vi "benchmark-tagContainer.vi"() -> (3 "write":dbl[](array[numeric])=[3.499321937561036e-05, 1.2534141540527342e-06, 6.518125534057617e-07, 1.403627395629883e-05, 0.00020125420093536383] caption="average" format="%#_6p")   [LabVIEW 2017]
uses:
  c133460f-0aec-4b14-aa01-684956f011bf.vi
  679e9543-87f0-4a91-8f0b-568c5a8b50fd.vi
  TagContainer/_Support/_NameCacher.vi
  TagContainer/_Support/_datatypeChecker.vi
  TagContainer/_Support/_Ref To DVR.vi
  <vilib>/Utility/Data Type/Get Type Information.vi
  <vilib>/Utility/error.llb/Trim Whitespace.vi
  TagContainer/TagContainer.lvlib
panel:
  out "error out":errorcluster
  in  "group name in (Untitled)":string="add changelock and globalchangetimestamp"
  out "length":i32=1170
  out "unit (ms)":cluster{dbl[]}[](graph)=[{[3.508806228637695e-05, 3.5092830657958984e-05, 3.508806228637695e-05, 3.509044647216797e-05, 3.509759902954102e-05, 3.5092830657958984e-05, 3.5092830657958984e-05, 3.509044647216797e-05, 3.5092830657958984e-05, 3.5092830657958984e-05, 3.509044647216797e-05, 3.509521484375e-05, 3.5092830657958984e-05, 3.508806228637695e-05, 3.509044647216797e-05, 3.5092830657958984e-05, 3.509044647216797e-05, 3.508806228637695e-05, 3.5092830657958984e-05, 3.5092830657958984e-05, 3.509521484375e-05, 3.5092830657958984e-05, 3.5092830657958984e-05, 3.508806228637695e-05, 3.509044647216797e-05, 3.5092830657958984e-05, 3.5092830657958984e-05, 3.5092830657958984e-05, 3.5092830657958984e-05, 3.5092830657958984e-05, 3.5092830657958984e-05, 3.5092830657958984e-05, 3.509044647216797e-05, 3.5092830657958984e-05, 3.509044647216797e-05, 3.509759902954102e-05, 3.509521484375e-05, 3.509521484375e-05, 3.5092830657958984e-05, 3.5092830657958984e-05, 3.5092830657958984e-05, 3.5092830657958984e-05, 3.5092830657958984e-05, 3.5092830657958984e-05, 3.5092830657958984e-05, 3.508806228637695e-05, 3.5092830657958984e-05, 3.5092830657958984e-05, 3.5092830657958984e-05, 3.007650375366211e-05, 3.5092830657958984e-05, 3.509044647216797e-05, 3.509044647216797e-05, 3.508806228637695e-05, 3.509044647216797e-05, 3.508806228637695e-05, 3.509044647216797e-05, 3.5092830657958984e-05, 3.509044647216797e-05, 3.508806228637695e-05, 3.5092830657958984e-05, 3.5092830657958984e-05, 3.509044647216797e-05, 3.509044647216797e-05, 3.5092830657958984e-05, 3.5092830657958984e-05, 3.5092830657958984e-05, 4.024505615234375e-05, 3.5092830657958984e-05, 3.5092830657958984e-05, 3.5092830657958984e-05, 3.5092830657958984e-05, 3.509044647216797e-05, 3.5092830657958984e-05, 3.509044647216797e-05, 3.5092830657958984e-05, 3.5092830657958984e-05, 3.5092830657958984e-05, 3.5092830657958984e-05, 3.008127212524414e-05, 3.0078887939453124e-05, 3.509044647216797e-05, 3.5092830657958984e-05, 3.509044647216797e-05, 3.5092830657958984e-05, 3.508806228637695e-05, 3.508806228637695e-05, 3.5092830657958984e-05, 3.509044647216797e-05, 3.509521484375e-05, 3.509521484375e-05, 3.509759902954102e-05, 3.5092830657958984e-05, 3.5092830657958984e-05, 3.508806228637695e-05, 3.509521484375e-05, 3.509759902954102e-05, 3.509044647216797e-05, 3.5092830657958984e-05, 3.5092830657958984e-05]}, {[0.0, 0.0, 0.0, 0.0, 0.0, 0.0, 0.0, 0.0, 0.0, 0.0, 0.0, 0.0, 0.0, 0.0, 0.0, 5.011558532714844e-06, 5.016326904296875e-06, 0.0, 0.0, 0.0, 0.0, 5.01394271850586e-06, 0.0, 0.0, 5.011558532714844e-06, 5.011558532714844e-06, 0.0, 0.0, 0.0, 0.0, 0.0, 5.016326904296875e-06, 0.0, 0.0, 0.0, 5.011558532714844e-06, 5.011558532714844e-06, 0.0, 5.016326904296875e-06, 0.0, 0.0, 5.011558532714844e-06, 0.0, 5.018711090087891e-06, 0.0, 0.0, 0.0, 0.0, 0.0, 5.016326904296875e-06, 5.016326904296875e-06, 0.0, 0.0, 0.0, 0.0, 0.0, 0.0, 5.016326904296875e-06, 0.0, 0.0, 5.011558532714844e-06, 0.0, 5.01394271850586e-06, 0.0, 0.0, 0.0, 0.0, 5.011558532714844e-06, 5.016326904296875e-06, 0.0, 5.011558532714844e-06, 5.011558532714844e-06, 0.0, 0.0, 0.0, 5.011558532714844e-06, 0.0, 0.0, 0.0, 5.016326904296875e-06, 5.01394271850586e-06, 0.0, 0.0, 5.01394271850586e-06, 0.0, 0.0, 0.0, 0.0, 0.0, 0.0, 5.0091743469238285e-06, 0.0, 0.0, 0.0, 0.0, 0.0, 0.0, 0.0, 0.0, 0.0]}, {[0.0, 0.0, 0.0, 0.0, 0.0, 0.0, 5.016326904296875e-06, 0.0, 0.0, 0.0, 0.0, 0.0, 5.016326904296875e-06, 0.0, 0.0, 0.0, 0.0, 5.01394271850586e-06, 0.0, 0.0, 0.0, 0.0, 0.0, 0.0, 0.0, 0.0, 5.016326904296875e-06, 0.0, 0.0, 0.0, 0.0, 0.0, 0.0, 0.0, 5.016326904296875e-06, 0.0, 0.0, 0.0, 0.0, 0.0, 0.0, 0.0, 0.0, 0.0, 0.0, 0.0, 0.0, 0.0, 5.011558532714844e-06, 0.0, 0.0, 0.0, 0.0, 0.0, 0.0, 5.016326904296875e-06, 0.0, 0.0, 0.0, 0.0, 0.0, 5.016326904296875e-06, 0.0, 0.0, 0.0, 0.0, 0.0, 0.0, 0.0, 0.0, 0.0, 0.0, 5.011558532714844e-06, 5.011558532714844e-06, 0.0, 0.0, 0.0, 0.0, 0.0, 0.0, 0.0, 5.0091743469238285e-06, 0.0, 0.0, 0.0, 0.0, 0.0, 0.0, 5.01394271850586e-06, 0.0, 0.0, 0.0, 0.0, 0.0, 0.0, 0.0, 5.011558532714844e-06, 0.0, 0.0, 0.0]}, {[0.0, 0.0, 5.016326904296875e-06, 5.01394271850586e-06, 0.0, 0.0, 0.0, 0.0, 5.011558532714844e-06, 5.016326904296875e-06, 5.01394271850586e-06, 5.011558532714844e-06, 0.0, 5.01394271850586e-06, 5.01394271850586e-06, 5.01394271850586e-06, 5.011558532714844e-06, 5.01394271850586e-06, 5.011558532714844e-06, 5.011558532714844e-06, 1.0023117065429687e-05, 5.01394271850586e-06, 5.011558532714844e-06, 5.016326904296875e-06, 5.016326904296875e-06, 5.011558532714844e-06, 5.011558532714844e-06, 1.0023117065429687e-05, 1.0023117065429687e-05, 1.0023117065429687e-05, 1.0023117065429687e-05, 5.011558532714844e-06, 1.0025501251220702e-05, 1.0023117065429687e-05, 5.011558532714844e-06, 1.0023117065429687e-05, 1.0025501251220702e-05, 1.0023117065429687e-05, 1.0023117065429687e-05, 1.5039443969726562e-05, 1.5039443969726562e-05, 1.002788543701172e-05, 1.5034675598144532e-05, 1.0020732879638672e-05, 1.5037059783935547e-05, 1.5039443969726562e-05, 1.5037059783935547e-05, 1.5039443969726562e-05, 1.0025501251220702e-05, 1.5039443969726562e-05, 1.0023117065429687e-05, 1.5037059783935547e-05, 1.5039443969726562e-05, 1.5041828155517579e-05, 2.0053386688232422e-05, 1.5041828155517579e-05, 1.5041828155517579e-05, 1.5034675598144532e-05, 1.5039443969726562e-05, 1.5039443969726562e-05, 1.5039443969726562e-05, 1.5034675598144532e-05, 1.5039443969726562e-05, 1.5041828155517579e-05, 2.0053386688232422e-05, 2.0051002502441405e-05, 2.0051002502441405e-05, 1.5056133270263672e-05, 1.5034675598144532e-05, 2.0053386688232422e-05, 2.0051002502441405e-05, 2.0051002502441405e-05, 2.0053386688232422e-05, 2.005577087402344e-05, 2.5064945220947265e-05, 2.0053386688232422e-05, 2.0051002502441405e-05, 2.0051002502441405e-05, 2.506256103515625e-05, 2.0051002502441405e-05, 2.0051002502441405e-05, 2.005577087402344e-05, 2.506732940673828e-05, 2.005577087402344e-05, 2.506256103515625e-05, 2.506732940673828e-05, 2.5069713592529298e-05, 2.506732940673828e-05, 2.506256103515625e-05, 2.5060176849365234e-05, 2.506732940673828e-05, 2.506256103515625e-05, 2.506256103515625e-05, 3.007650375366211e-05, 3.008127212524414e-05, 2.5064945220947265e-05, 2.506256103515625e-05, 2.5064945220947265e-05, 3.008127212524414e-05, 3.0074119567871094e-05]}, {[5.011558532714844e-06, 1.002788543701172e-05, 1.002788543701172e-05, 1.5034675598144532e-05, 2.506256103515625e-05, 2.506256103515625e-05, 3.007650375366211e-05, 3.5092830657958984e-05, 3.509044647216797e-05, 4.010438919067383e-05, 4.511594772338867e-05, 4.511594772338867e-05, 5.514621734619141e-05, 5.514383316040039e-05, 6.015777587890625e-05, 6.0155391693115235e-05, 6.517410278320313e-05, 7.018327713012695e-05, 8.021116256713867e-05, 8.020877838134766e-05, 8.020877838134766e-05, 9.023427963256837e-05, 9.525299072265625e-05, 9.524822235107422e-05, 0.00010048389434814453, 0.00010527610778808594, 0.00011028766632080078, 0.00011029243469238282, 0.00011530399322509766, 0.0001203155517578125, 0.0001203155517578125, 0.00013034105300903322, 0.00013535499572753907, 0.00013535737991333008, 0.0001403641700744629, 0.00014036893844604492, 0.0001503920555114746, 0.0001503920555114746, 0.0001554083824157715, 0.00015540361404418944, 0.00016041994094848633, 0.00017044782638549804, 0.00017044782638549804, 0.00018047094345092775, 0.00018047571182250977, 0.0001854872703552246, 0.00019049882888793945, 0.00019049882888793945, 0.00020052671432495118, 0.00019550800323486328, 0.00020554065704345704, 0.00020554065704345704, 0.00021055221557617188, 0.00021556377410888672, 0.00021556615829467773, 0.00022057533264160155, 0.0002255868911743164, 0.0002306056022644043, 0.000240633487701416, 0.000240631103515625, 0.00024062871932983398, 0.00024564504623413085, 0.0002506566047668457, 0.0002556657791137695, 0.00025567054748535154, 0.00026067972183227536, 0.0002656960487365723, 0.0002706313133239746, 0.000275723934173584, 0.00027571916580200196, 0.000275723934173584, 0.00028073787689208984, 0.00028574705123901367, 0.0002907609939575195, 0.0002957749366760254, 0.0003007864952087402, 0.00030580043792724607, 0.000310816764831543, 0.0003158235549926758, 0.0003184247016906738, 0.0003208446502685547, 0.00033086299896240235, 0.00033086538314819336, 0.00034089088439941405, 0.00034089326858520507, 0.0003408956527709961, 0.00035091400146484373, 0.00035092115402221677, 0.00035593271255493166, 0.00035593271255493166, 0.0003609395027160645, 0.00036596059799194337, 0.0003709721565246582, 0.0003709745407104492, 0.0003809952735900879, 0.00038600683212280273, 0.0003910255432128906, 0.0003910231590270996, 0.00039603471755981443, 0.00039603710174560545]}]
  out "outside":i32=99
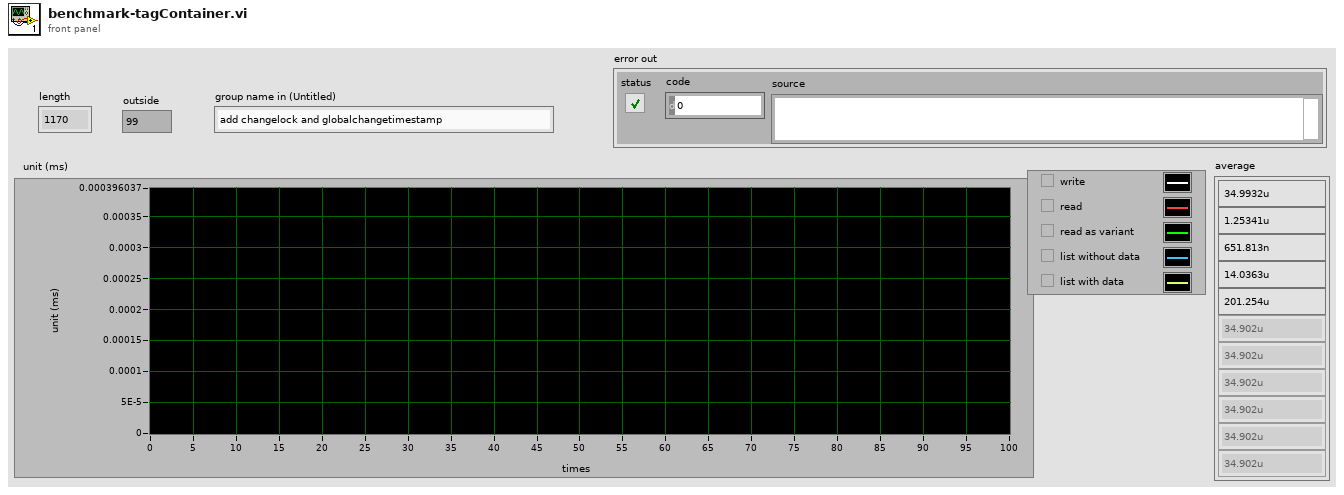
[diagram p1: front panel]
types:
  T1 = enum16{"open", "open or create", "create or replace", "create", "open (read-only)"}
  T2 = cluster{"error constant":errorcluster, "error constant 2":errorcluster, "error constant 3":errorcluster, "error constant 4":errorcluster, "error constant 5":errorcluster, "error constant 6":errorcluster, "error constant 7":errorcluster, "error constant 8":errorcluster, "error constant 9":errorcluster, "error constant 10":errorcluster, "error constant 11":errorcluster, "error constant 12":errorcluster, "error constant 13":errorcluster, "error constant 14":errorcluster, "error constant 15":errorcluster, "error constant 16":errorcluster, "error constant 17":errorcluster, "error constant 18":errorcluster, "error constant 19":errorcluster, "error constant 20":errorcluster, "error constant 21":errorcluster, "error constant 22":errorcluster, "error constant 23":errorcluster, "error constant 24":errorcluster, "error constant 25":errorcluster, "error constant 26":errorcluster, "error constant 27":errorcluster, "error constant 28":errorcluster, "error constant 29":errorcluster, "error constant 30":errorcluster, "error constant 31":errorcluster, "error constant 32":errorcluster, "error constant 33":errorcluster, "error constant 34":errorcluster, "error constant 35":errorcluster, "error constant 36":errorcluster, "error constant 37":errorcluster, "error constant 38":errorcluster, "error constant 39":errorcluster, "error constant 40":errorcluster, "error constant 41":errorcluster, "error constant 42":errorcluster, "error constant 43":errorcluster, "error constant 44":errorcluster, "error constant 45":errorcluster, "error constant 46":errorcluster, "error constant 47":errorcluster, "error constant 48":errorcluster, "error constant 49":errorcluster, "error constant 50":errorcluster, "error constant 51":errorcluster, "error constant 52":errorcluster, "error constant 53":errorcluster, "error constant 54":errorcluster, "error constant 55":errorcluster, "error constant 56":errorcluster, "error constant 57":errorcluster, "error constant 58":errorcluster, "error constant 59":errorcluster, "error constant 60":errorcluster, "error constant 61":errorcluster, "error constant 62":errorcluster, "error constant 63":errorcluster, "error constant 64":errorcluster, "error constant 65":errorcluster, cluster{"error constant":errorcluster, "error constant 2":errorcluster, "error constant 3":errorcluster, "error constant 4":errorcluster, "error constant 5":errorcluster, "error constant 6":errorcluster, "error constant 7":errorcluster, "error constant 8":errorcluster, "error constant 9":errorcluster, "error constant 10":errorcluster, "error constant 11":errorcluster, "error constant 12":errorcluster, "error constant 13":errorcluster, "error constant 14":errorcluster, "error constant 15":errorcluster, "error constant 16":errorcluster, "error constant 17":errorcluster, "error constant 18":errorcluster, "error constant 19":errorcluster, "error constant 20":errorcluster, "error constant 21":errorcluster, "error constant 22":errorcluster, "error constant 23":errorcluster, "error constant 24":errorcluster, "error constant 25":errorcluster, "error constant 26":errorcluster, "error constant 27":errorcluster, "error constant 28":errorcluster, "error constant 29":errorcluster, "error constant 30":errorcluster, "error constant 31":errorcluster, "error constant 32":errorcluster, "error constant 33":errorcluster, "error constant 34":errorcluster, "error constant 35":errorcluster, "error constant 36":errorcluster, "error constant 37":errorcluster, "error constant 38":errorcluster, "error constant 39":errorcluster, "error constant 40":errorcluster, "error constant 41":errorcluster, "error constant 42":errorcluster, "error constant 43":errorcluster, "error constant 44":errorcluster, "error constant 45":errorcluster, "error constant 46":errorcluster, "error constant 47":errorcluster, "error constant 48":errorcluster, "error constant 49":errorcluster, "error constant 50":errorcluster, "error constant 51":errorcluster, "error constant 52":errorcluster, "error constant 53":errorcluster, "error constant 54":errorcluster, "error constant 55":errorcluster, "error constant 56":errorcluster, "error constant 57":errorcluster, "error constant 58":errorcluster, "error constant 59":errorcluster, "error constant 60":errorcluster, "error constant 61":errorcluster, "error constant 62":errorcluster, "error constant 63":errorcluster, "error constant 64":errorcluster, "error constant 65":errorcluster}}
  T3 = typedef "TagContainer.lvlib/TagContainer.ctl" = refnum<k1>
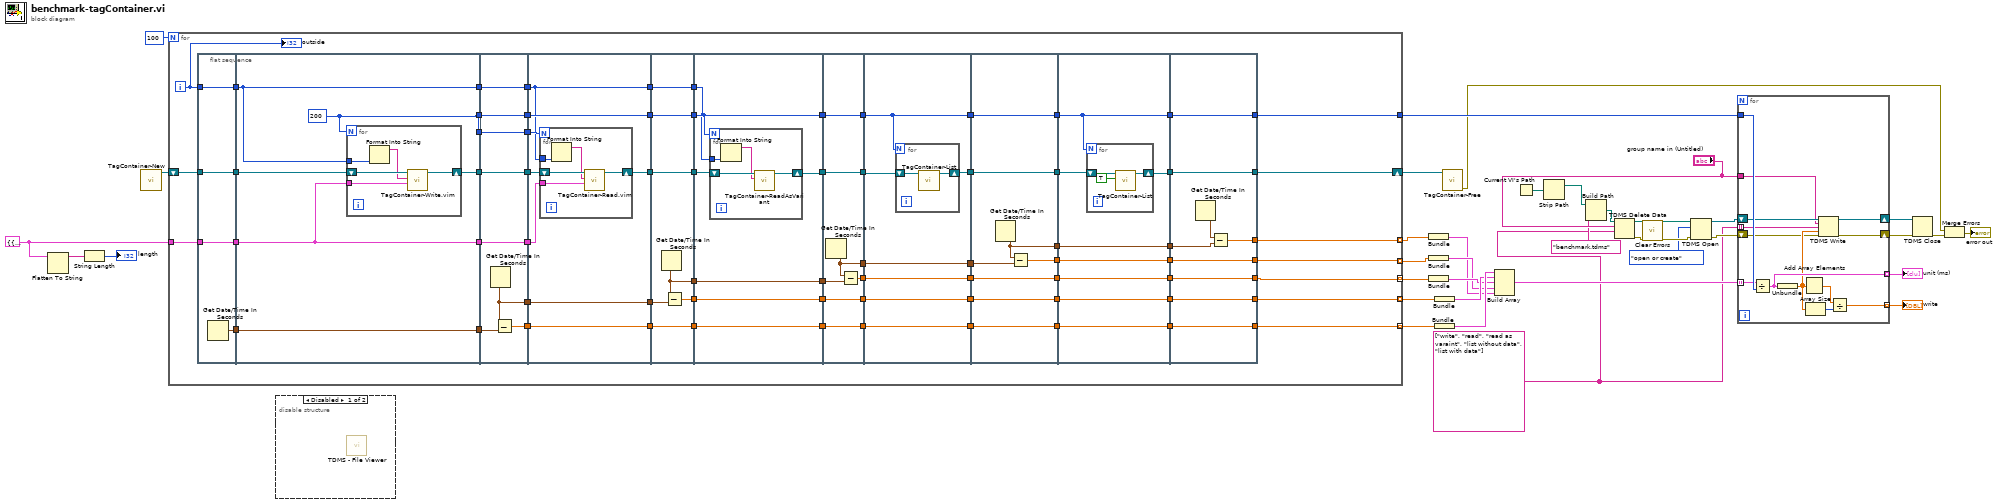
[diagram p0: block diagram]
diagram:
  w3 = string[] ["write", "read", "read as varaint", "list without data", "list with data"]
  w33 = T2 {"error constant"={"status"=FALSE, "code"=0, "source"=""}, "error constant 2"={"status"=FALSE, "code"=0, "source"=""}, "error constant 3"={"status"=FALSE, "code"=0, "source"=""}, "error constant 4"={"status"=FALSE, "code"=0, "source"=""}, "error constant 5"={"status"=FALSE, "code"=0, "source"=""}, "error constant 6"={"status"=FALSE, "code"=0, "source"=""}, "error constant 7"={"status"=FALSE, "code"=0, "source"=""}, "error constant 8"={"status"=FALSE, "code"=0, "source"=""}, "error constant 9"={"status"=FALSE, "code"=0, "source"=""}, "error constant 10"={"status"=FALSE, "code"=0, "source"=""}, "error constant 11"={"status"=FALSE, "code"=0, "source"=""}, "error constant 12"={"status"=FALSE, "code"=0, "source"=""}, "error constant 13"={"status"=FALSE, "code"=0, "source"=""}, "error constant 14"={"status"=FALSE, "code"=0, "source"=""}, "error constant 15"={"status"=FALSE, "code"=0, "source"=""}, "error constant 16"={"status"=FALSE, "code"=0, "source"=""}, "error constant 17"={"status"=FALSE, "code"=0, "source"=""}, "error constant 18"={"status"=FALSE, "code"=0, "source"=""}, "error constant 19"={"status"=FALSE, "code"=0, "source"=""}, "error constant 20"={"status"=FALSE, "code"=0, "source"=""}, "error constant 21"={"status"=FALSE, "code"=0, "source"=""}, "error constant 22"={"status"=FALSE, "code"=0, "source"=""}, "error constant 23"={"status"=FALSE, "code"=0, "source"=""}, "error constant 24"={"status"=FALSE, "code"=0, "source"=""}, "error constant 25"={"status"=FALSE, "code"=0, "source"=""}, "error constant 26"={"status"=FALSE, "code"=0, "source"=""}, "error constant 27"={"status"=FALSE, "code"=0, "source"=""}, "error constant 28"={"status"=FALSE, "code"=0, "source"=""}, "error constant 29"={"status"=FALSE, "code"=0, "source"=""}, "error constant 30"={"status"=FALSE, "code"=0, "source"=""}, "error constant 31"={"status"=FALSE, "code"=0, "source"=""}, "error constant 32"={"status"=FALSE, "code"=0, "source"=""}, "error constant 33"={"status"=FALSE, "code"=0, "source"=""}, "error constant 34"={"status"=FALSE, "code"=0, "source"=""}, "error constant 35"={"status"=FALSE, "code"=0, "source"=""}, "error constant 36"={"status"=FALSE, "code"=0, "source"=""}, "error constant 37"={"status"=FALSE, "code"=0, "source"=""}, "error constant 38"={"status"=FALSE, "code"=0, "source"=""}, "error constant 39"={"status"=FALSE, "code"=0, "source"=""}, "error constant 40"={"status"=FALSE, "code"=0, "source"=""}, "error constant 41"={"status"=FALSE, "code"=0, "source"=""}, "error constant 42"={"status"=FALSE, "code"=0, "source"=""}, "error constant 43"={"status"=FALSE, "code"=0, "source"=""}, "error constant 44"={"status"=FALSE, "code"=0, "source"=""}, "error constant 45"={"status"=FALSE, "code"=0, "source"=""}, "error constant 46"={"status"=FALSE, "code"=0, "source"=""}, "error constant 47"={"status"=FALSE, "code"=0, "source"=""}, "error constant 48"={"status"=FALSE, "code"=0, "source"=""}, "error constant 49"={"status"=FALSE, "code"=0, "source"=""}, "error constant 50"={"status"=FALSE, "code"=0, "source"=""}, "error constant 51"={"status"=FALSE, "code"=0, "source"=""}, "error constant 52"={"status"=FALSE, "code"=0, "source"=""}, "error constant 53"={"status"=FALSE, "code"=0, "source"=""}, "error constant 54"={"status"=FALSE, "code"=0, "source"=""}, "error constant 55"={"status"=FALSE, "code"=0, "source"=""}, "error constant 56"={"status"=FALSE, "code"=0, "source"=""}, "error constant 57"={"status"=FALSE, "code"=0, "source"=""}, "error constant 58"={"status"=FALSE, "code"=0, "source"=""}, "error constant 59"={"status"=FALSE, "code"=0, "source"=""}, "error constant 60"={"status"=FALSE, "code"=0, "source"=""}, "error constant 61"={"status"=FALSE, "code"=0, "source"=""}, "error constant 62"={"status"=FALSE, "code"=0, "source"=""}, "error constant 63"={"status"=FALSE, "code"=0, "source"=""}, "error constant 64"={"status"=FALSE, "code"=0, "source"=""}, "error constant 65"={"status"=FALSE, "code"=0, "source"=""}, {"error constant"={"status"=FALSE, "code"=0, "source"=""}, "error constant 2"={"status"=FALSE, "code"=0, "source"=""}, "error constant 3"={"status"=FALSE, "code"=0, "source"=""}, "error constant 4"={"status"=FALSE, "code"=0, "source"=""}, "error constant 5"={"status"=FALSE, "code"=0, "source"=""}, "error constant 6"={"status"=FALSE, "code"=0, "source"=""}, "error constant 7"={"status"=FALSE, "code"=0, "source"=""}, "error constant 8"={"status"=FALSE, "code"=0, "source"=""}, "error constant 9"={"status"=FALSE, "code"=0, "source"=""}, "error constant 10"={"status"=FALSE, "code"=0, "source"=""}, "error constant 11"={"status"=FALSE, "code"=0, "source"=""}, "error constant 12"={"status"=FALSE, "code"=0, "source"=""}, "error constant 13"={"status"=FALSE, "code"=0, "source"=""}, "error constant 14"={"status"=FALSE, "code"=0, "source"=""}, "error constant 15"={"status"=FALSE, "code"=0, "source"=""}, "error constant 16"={"status"=FALSE, "code"=0, "source"=""}, "error constant 17"={"status"=FALSE, "code"=0, "source"=""}, "error constant 18"={"status"=FALSE, "code"=0, "source"=""}, "error constant 19"={"status"=FALSE, "code"=0, "source"=""}, "error constant 20"={"status"=FALSE, "code"=0, "source"=""}, "error constant 21"={"status"=FALSE, "code"=0, "source"=""}, "error constant 22"={"status"=FALSE, "code"=0, "source"=""}, "error constant 23"={"status"=FALSE, "code"=0, "source"=""}, "error constant 24"={"status"=FALSE, "code"=0, "source"=""}, "error constant 25"={"status"=FALSE, "code"=0, "source"=""}, "error constant 26"={"status"=FALSE, "code"=0, "source"=""}, "error constant 27"={"status"=FALSE, "code"=0, "source"=""}, "error constant 28"={"status"=FALSE, "code"=0, "source"=""}, "error constant 29"={"status"=FALSE, "code"=0, "source"=""}, "error constant 30"={"status"=FALSE, "code"=0, "source"=""}, "error constant 31"={"status"=FALSE, "code"=0, "source"=""}, "error constant 32"={"status"=FALSE, "code"=0, "source"=""}, "error constant 33"={"status"=FALSE, "code"=0, "source"=""}, "error constant 34"={"status"=FALSE, "code"=0, "source"=""}, "error constant 35"={"status"=FALSE, "code"=0, "source"=""}, "error constant 36"={"status"=FALSE, "code"=0, "source"=""}, "error constant 37"={"status"=FALSE, "code"=0, "source"=""}, "error constant 38"={"status"=FALSE, "code"=0, "source"=""}, "error constant 39"={"status"=FALSE, "code"=0, "source"=""}, "error constant 40"={"status"=FALSE, "code"=0, "source"=""}, "error constant 41"={"status"=FALSE, "code"=0, "source"=""}, "error constant 42"={"status"=FALSE, "code"=0, "source"=""}, "error constant 43"={"status"=FALSE, "code"=0, "source"=""}, "error constant 44"={"status"=FALSE, "code"=0, "source"=""}, "error constant 45"={"status"=FALSE, "code"=0, "source"=""}, "error constant 46"={"status"=FALSE, "code"=0, "source"=""}, "error constant 47"={"status"=FALSE, "code"=0, "source"=""}, "error constant 48"={"status"=FALSE, "code"=0, "source"=""}, "error constant 49"={"status"=FALSE, "code"=0, "source"=""}, "error constant 50"={"status"=FALSE, "code"=0, "source"=""}, "error constant 51"={"status"=FALSE, "code"=0, "source"=""}, "error constant 52"={"status"=FALSE, "code"=0, "source"=""}, "error constant 53"={"status"=FALSE, "code"=0, "source"=""}, "error constant 54"={"status"=FALSE, "code"=0, "source"=""}, "error constant 55"={"status"=FALSE, "code"=0, "source"=""}, "error constant 56"={"status"=FALSE, "code"=0, "source"=""}, "error constant 57"={"status"=FALSE, "code"=0, "source"=""}, "error constant 58"={"status"=FALSE, "code"=0, "source"=""}, "error constant 59"={"status"=FALSE, "code"=0, "source"=""}, "error constant 60"={"status"=FALSE, "code"=0, "source"=""}, "error constant 61"={"status"=FALSE, "code"=0, "source"=""}, "error constant 62"={"status"=FALSE, "code"=0, "source"=""}, "error constant 63"={"status"=FALSE, "code"=0, "source"=""}, "error constant 64"={"status"=FALSE, "code"=0, "source"=""}, "error constant 65"={"status"=FALSE, "code"=0, "source"=""}}}
  n1 = Flatten To String(anything=w33) -> (data string=w32:string)  [unwired: 3 in, 2 out]
  n2 = String Length(string=w32) -> (length=→"length":i32)
  n3 = call "TagContainer-New.vi"() -> ("TagContainer"=w35:T3)  [unwired: 10 in, 1 out]
  n4 = for {
    N: 100 -> [_]
    tunnel: [w104] -> w27 mode=indexing
    tunnel: [w103] -> w29
    tunnel: w33 -> [w93]
    shift-right: [w91] -> w34
    shift-left: w35 -> [w92]
    tunnel: [w86] -> w28 mode=indexing
    tunnel: [w73] -> w25 mode=indexing
    tunnel: [w39] -> w24 mode=indexing
    tunnel: [w38] -> w23 mode=indexing
    i -> [w101]
    n5 = flat-sequence {
      tunnel: [w110] -> w106
      tunnel: [w109] -> w96
      tunnel: [w108] -> w95
      tunnel: [w107] -> w94
      tunnel: w92 -> [w109]
      tunnel: w93 -> [w108]
      tunnel: w101 -> [w107]
      tunnel: w106 -> [w116]
      tunnel: [w116] -> w105
      tunnel: [w112] -> w102
      tunnel: [w114] -> w97
      tunnel: w96 -> [w115]
      tunnel: w95 -> [w111]
      tunnel: w94 -> [w113]
      tunnel: [w112] -> w84
      tunnel: [w113] -> w81
      tunnel: [w111] -> w79
      tunnel: w105 -> [w126]
      tunnel: w102 -> [w128]
      tunnel: [w129] -> w100
      tunnel: [w128] -> w99
      tunnel: [w127] -> w98
      tunnel: w97 -> [w127]
      tunnel: [w122] -> w88
      tunnel: w84 -> [w125]
      tunnel: [w125] -> w83
      tunnel: [w124] -> w82
      tunnel: w81 -> [w124]
      tunnel: [w123] -> w80
      tunnel: w79 -> [w123]
      tunnel: w100 -> [w137]
      tunnel: w99 -> [w136]
      tunnel: w98 -> [w134]
      tunnel: [w137] -> w90
      tunnel: [w136] -> w89
      tunnel: w88 -> [w135]
      tunnel: [w135] -> w87
      tunnel: [w133] -> w85
      tunnel: w83 -> [w132]
      tunnel: w82 -> [w130]
      tunnel: w80 -> [w131]
      tunnel: [w130] -> w72
      tunnel: w90 -> [w149]
      tunnel: w89 -> [w146]
      tunnel: w87 -> [w148]
      tunnel: w85 -> [w144]
      tunnel: [w149] -> w71
      tunnel: [w146] -> w70
      tunnel: [w147] -> w69
      tunnel: [w145] -> w68
      tunnel: w72 -> [w145]
      tunnel: [w144] -> w67
      tunnel: [w143] -> w66
      tunnel: w71 -> [w156]
      tunnel: w70 -> [w153]
      tunnel: w69 -> [w155]
      tunnel: [w156] -> w78
      tunnel: [w153] -> w77
      tunnel: [w154] -> w76
      tunnel: [w155] -> w75
      tunnel: [w150] -> w74
      tunnel: w68 -> [w152]
      tunnel: w67 -> [w151]
      tunnel: w66 -> [w150]
      tunnel: w78 -> [w167]
      tunnel: w77 -> [w166]
      tunnel: w76 -> [w165]
      tunnel: w75 -> [w164]
      tunnel: w74 -> [w163]
      tunnel: [w167] -> w65
      tunnel: [w166] -> w64
      tunnel: [w165] -> w63
      tunnel: [w164] -> w62
      tunnel: [w162] -> w61
      tunnel: [w161] -> w55
      tunnel: w65 -> [w174]
      tunnel: w64 -> [w168]
      tunnel: w63 -> [w171]
      tunnel: w62 -> [w173]
      tunnel: w61 -> [w172]
      tunnel: [w174] -> w60
      tunnel: [w168] -> w59
      tunnel: [w170] -> w58
      tunnel: [w173] -> w57
      tunnel: [w172] -> w56
      tunnel: w55 -> [w169]
      tunnel: [w169] -> w54
      tunnel: w60 -> [w184]
      tunnel: w59 -> [w183]
      tunnel: w58 -> [w182]
      tunnel: w57 -> [w181]
      tunnel: w56 -> [w180]
      tunnel: w54 -> [w179]
      tunnel: [w184] -> w53
      tunnel: [w183] -> w52
      tunnel: [w182] -> w51
      tunnel: [w181] -> w50
      tunnel: [w180] -> w49
      tunnel: [w178] -> w48
      tunnel: [w177] -> w41
      tunnel: w53 -> [w192]
      tunnel: w52 -> [w185]
      tunnel: w51 -> [w188]
      tunnel: w50 -> [w191]
      tunnel: w49 -> [w190]
      tunnel: w48 -> [w189]
      tunnel: [w192] -> w47
      tunnel: [w185] -> w46
      tunnel: [w187] -> w45
      tunnel: [w191] -> w44
      tunnel: [w190] -> w43
      tunnel: [w189] -> w42
      tunnel: w41 -> [w186]
      tunnel: [w186] -> w40
      tunnel: [w199] -> w38
      tunnel: [w200] -> w73
      tunnel: [w201] -> w86
      tunnel: [w202] -> w91
      tunnel: [w203] -> w103
      tunnel: [w204] -> w104
      tunnel: w47 -> [w204]
      tunnel: w46 -> [w203]
      tunnel: w45 -> [w202]
      tunnel: w44 -> [w201]
      tunnel: w43 -> [w200]
      tunnel: w42 -> [w199]
      tunnel: w40 -> [w197]
      tunnel: [w196] -> w39
      frame #0 {
        n6 = Get Date/Time In Seconds() -> (seconds since 1Jan1904=w110:timestamp)
      }
      frame #1 {
        w112 = 200
        n7 = for {
          N: w112 -> [_]
          tunnel: w111 -> [w119]
          tunnel: w113 -> [w118]
          shift-right: [w120] -> w114
          shift-left: w115 -> [w121]
          n8 = Format Into String(w118) -> (resulting string=w117:string)  [unwired: 3 in, 1 out]
          n9 = call "TagContainer-Write.vim"("Value"=w119, "name"=w117, "TagContainer"=w121) -> ("TagContainer(dup)"=w120:T3)  [unwired: 7 in, 1 out]
        }
      }
      frame #2 {
        n10 = Get Date/Time In Seconds() -> (seconds since 1Jan1904=w122:timestamp)
        n11 = Subtract(x=w122, y=w126) -> (x-y=w129:dbl)
      }
      frame #3 {
        n12 = for {
          N: w132 -> [_]
          shift-right: [w141] -> w133
          shift-left: w134 -> [w142]
          tunnel: w130 -> [w139]
          tunnel: w131 -> [w138]
          n13 = Format Into String(w139) -> (resulting string=w140:string)  [unwired: 3 in, 1 out]
          n14 = call "TagContainer-Read.vim"("Type"=w138, "name"=w140, "TagContainer"=w142) -> ("TagContainer(dup)"=w141:T3)  [unwired: 3 in, 5 out]
        }
      }
      frame #4 {
        n15 = Get Date/Time In Seconds() -> (seconds since 1Jan1904=w143:timestamp)
        n16 = Subtract(x=w143, y=w148) -> (x-y=w147:dbl)
      }
      frame #5 {
        n17 = for {
          N: w153 -> [_]
          shift-right: [w159] -> w154
          shift-left: w151 -> [w160]
          tunnel: w152 -> [w157]
          n18 = Format Into String(w157) -> (resulting string=w158:string)  [unwired: 3 in, 1 out]
          n19 = call "TagContainer-ReadAsVariant.vi"("name"=w158, "TagContainer"=w160) -> ("TagContainer(dup)"=w159:T3)  [unwired: 4 in, 5 out]
        }
      }
      frame #6 {
        n20 = Get Date/Time In Seconds() -> (seconds since 1Jan1904=w161:timestamp)
        n21 = Subtract(x=w161, y=w163) -> (x-y=w162:dbl)
      }
      frame #7 {
        n22 = for {
          N: w168 -> [_]
          shift-right: [w175] -> w170
          shift-left: w171 -> [w176]
          n23 = call "TagContainer-List.vi"("TagContainer"=w176) -> ("TagContainer(dup)"=w175:T3)  [unwired: 7 in, 3 out]
        }
      }
      frame #8 {
        n24 = Get Date/Time In Seconds() -> (seconds since 1Jan1904=w177:timestamp)
        n25 = Subtract(x=w177, y=w179) -> (x-y=w178:dbl)
      }
      frame #9 {
        n26 = for {
          N: w185 -> [_]
          shift-right: [w194] -> w187
          shift-left: w188 -> [w195]
          n27 = call "TagContainer-List.vi"("with Data?(F)"=TRUE, "TagContainer"=w195) -> ("TagContainer(dup)"=w194:T3)  [unwired: 6 in, 3 out]
        }
      }
      frame #10 {
        n28 = Get Date/Time In Seconds() -> (seconds since 1Jan1904=w198:timestamp)
        n29 = Subtract(x=w198, y=w197) -> (x-y=w196:dbl)
      }
    }
    "outside" <- w101
  }
  n30 = disable-structure shown="Disabled" {
    frame Disabled {
      n31 = call <vilib>:"TDMS - File Viewer.vi"() -> ()  [unwired: 6 in, 2 out]
    }
    frame Enabled {
    }
  }
  n32 = Bundle(w24) -> (w18:cluster{dbl[]})  [unwired: 1 in]
  n33 = Bundle(w23) -> (w19:cluster{dbl[]})  [unwired: 1 in]
  n34 = Bundle(w25) -> (w20:cluster{dbl[]})  [unwired: 1 in]
  n35 = Bundle(w28) -> (w21:cluster{dbl[]})  [unwired: 1 in]
  n36 = Bundle(w27) -> (w22:cluster{dbl[]})  [unwired: 1 in]
  n37 = call "TagContainer-Free.vi"("TagContainer"=w34) -> ("error out"=w5:errorcluster)  [unwired: 10 in]
  n38 = Build Array(w22, w21, w20, w19, w18) -> (w26:cluster{dbl[]}[])
  n39 = Current VI's Path() -> (path=w2:path)
  n40 = Strip Path(path=w2) -> (stripped path=w1:path)  [unwired: 1 out]
  n41 = Build Path(base path=w1, name or relative path="benchmark.tdms") -> (appended path=w10:path)
  n42 = TDMS Delete Data(9:w3, 10:"group name in (Untitled)", 11:w10) -> (0:w12:errorcluster, 3:w11:path)  [unwired: 4 in]
  n43 = call <vilib>:"Clear Errors.vi"("error in (no error)"=w12) -> ("error out"=w8:errorcluster)  [unwired: 5 in, 1 out]
  n44 = TDMS Open(8:w8, 10:T1."open or create" ("operation (0:open)"), 11:w11) -> (0:w15:errorcluster, 3:w14:refnum<k34>)  [unwired: 4 in]
  n45 = for {
    tunnel: [w217] -> w31 mode=indexing
    tunnel: [w212] -> w30 mode=indexing
    tunnel: w29 -> [w214]
    tunnel: w26 -> [w213] mode=indexing
    shift-right: [w210] -> w17
    shift-left: w14 -> [w209]
    shift-right: [w208] -> w16
    shift-left: w15 -> [w207]
    tunnel: w3 -> [w206] mode=indexing
    tunnel: "group name in (Untitled)" -> [w205]
    n46 = Divide(x=w213, y=w214) -> (x/y=w212:cluster{dbl[]})
    n47 = Unbundle(w212) -> (w211:dbl[])
    n48 = Add Array Elements(numeric array=w211) -> (sum=w216:dbl)
    n49 = Array Size(array=w211) -> (size(s)=w215:i32)
    n50 = TDMS Write(0:w209, 5:w205, 7:w206, 9:w211, 11:w207) -> (4:w210:refnum<k34>, 15:w208:errorcluster)  [unwired: 1 in, 2 out]
    n51 = Divide(x=w216, y=w215) -> (x/y=w217:dbl)
  }
  "unit (ms)" <- w30
  "write" <- w31
  n52 = TDMS Close(8:w16, 11:w17) -> (0:w6:errorcluster)  [unwired: 1 out]
  n53 = Merge Errors(w5, w6) -> (→"error out":errorcluster)
